vi "Image Display_Set Colot Palette.vi"(5 "Image High Color":u32(colorbox)=16777216, 7 "Image Low Color":u32(colorbox)=16777216, 8 "Error In":errorcluster, 9 "Image Display Range":cluster{"Min Value":dbl, "Max Value":dbl}={"Min Value"=nan, "Max Value"=nan}, 10 "Image Display Palette Information":T1 {"Palette Type" items=["Grayscale", "Binary", "Gradient", "Rainbow", "Temperature", "User Defined", "Binary 16 Bit", "Gradient 16 Bit", "Rainbow 16 Bit", "Temperature 16 Bit", "User Defined 16 Bit"]}, 11 "Display Image Control Refnum":T3) -> (0 "Error Out":errorcluster)   [LabVIEW 2019]
uses:
  Image Control Refnum.ctl
  Image Display Palette Information.ctl
  Image Display Palette Type.ctl
panel:
  out "Image Low Color (U32)":u32
  out "Image High Color (U32)":u32
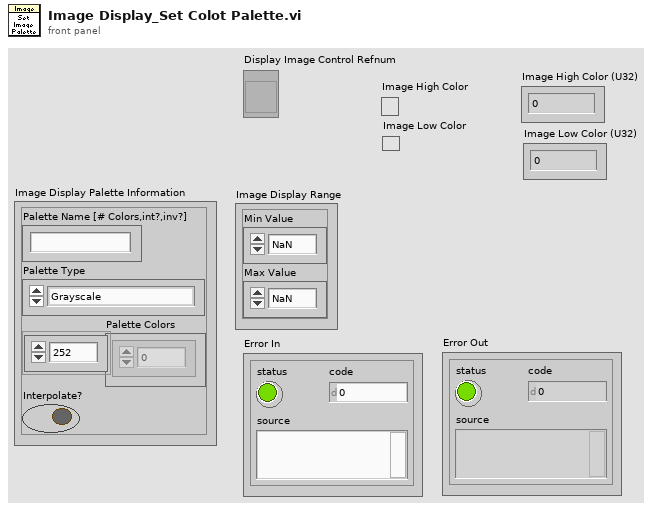
[diagram p1: front panel]
types:
  T1 = typedef "Image Display Palette Information.ctl" = cluster{"Palette Name [# Colors,int?,inv?]":string, "Palette Type":T2, "Palette Colors":u32[], "Interpolate?":bool}
  T2 = typedef "Image Display Palette Type.ctl" = u32
  T3 = typedef "Image Control Refnum.ctl" = refnum<vi>
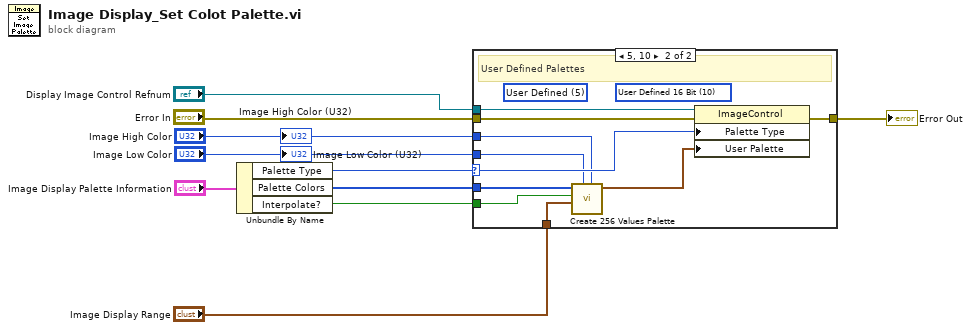
[diagram p0: block diagram]
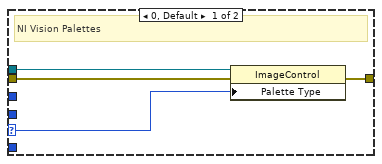
[diagram p2: hidden frame]
diagram:
  n1 = Unbundle By Name("Image Display Palette Information") -> ("Palette Type"=w5:T2, "Palette Colors"=w4:u32[], "Interpolate?"=w3:bool)
  n2 = case shown="5, 10" w5 {
    selector: w5 -> [w14 w24]
    tunnel: "Display Image Control Refnum" -> [w13 w23]
    tunnel: "Error In" -> [w12 w22]
    tunnel: [w11 w21] -> w8
    tunnel: "Image Display Range" -> [_ w18]
    tunnel: w4 -> [_ w19]
    tunnel: w3 -> [_ w17]
    tunnel: "Image High Color" -> [_ w16]
    tunnel: "Image Low Color" -> [_ w15]
    frame 0, Default {
      # "NI Vision Palettes"
      n3 = property class="ImageControl"(reference=w13, error in=w12, "Palette Type"=w14) -> (error out=w11:errorcluster)  [unwired: 1 out]
    }
    frame 5, 10 {
      (unwired) T2 10 items=["Grayscale", "Binary", "Gradient", "Rainbow", "Temperature", "User Defined", "Binary 16 Bit", "Gradient 16 Bit", "Rainbow 16 Bit", "Temperature 16 Bit", "User Defined 16 Bit"] ("Palette Type")
      (unwired) T2 5 items=["Grayscale", "Binary", "Gradient", "Rainbow", "Temperature", "User Defined", "Binary 16 Bit", "Gradient 16 Bit", "Rainbow 16 Bit", "Temperature 16 Bit", "User Defined 16 Bit"] ("Palette Type")
      # "User Defined Palettes"
      n4 = call "Create 256 Values Palette.vi"("Image High Color"=w16, "Image Low Color"=w15, "Source Image Display Range"=w18, "Interpolate?"=w17, "Palette Colors in"=w19) -> ("1D Color value array"=w20:cluster{"Red":u8, "Green":u8, "Blue":u8}[])  [unwired: 4 in, 2 out]
      n5 = property class="ImageControl"(reference=w23, error in=w22, "Palette Type"=w24, "User Palette"=w20) -> (error out=w21:errorcluster)  [unwired: 1 out]
    }
  }
  "Error Out" <- w8
  "Image High Color (U32)" <- "Image High Color"
  "Image Low Color (U32)" <- "Image Low Color"
